vi "OnlyOpenTheseValves_CMD.vi"(11 "Valve List":u16[](array[numeric])) -> (3 "Valve Comand":T1)   [LabVIEW 2016]
panel:
  in  "Flowboard":enum16{"A", "B", "C"}(ring)
  in  "Channel":enum16{"1", "2", "3", "4", "5", "6", "7", "8"}(ring)
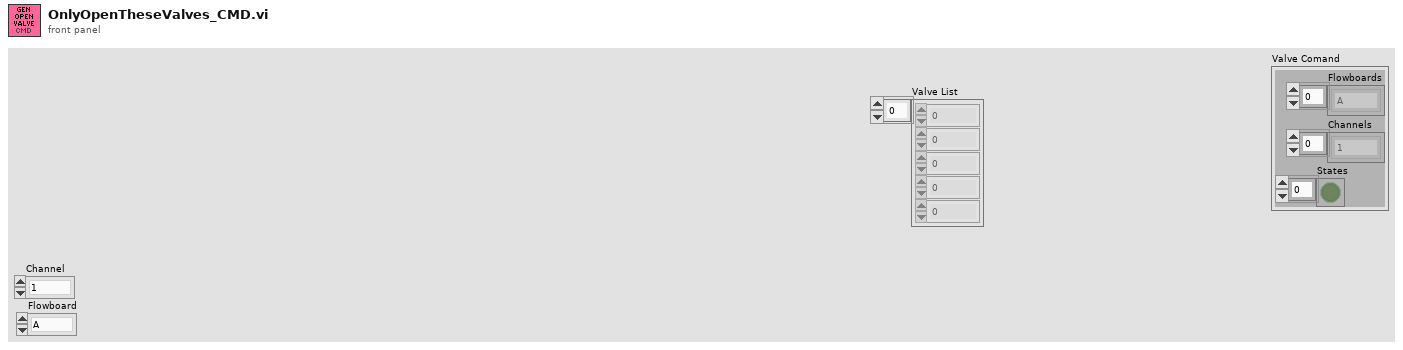
[diagram p1: front panel]
types:
  T1 = cluster{"Flowboards":enum16{"A", "B", "C"}[], "Channels":enum16{"1", "2", "3", "4", "5", "6", "7", "8"}[], "States":bool[]}
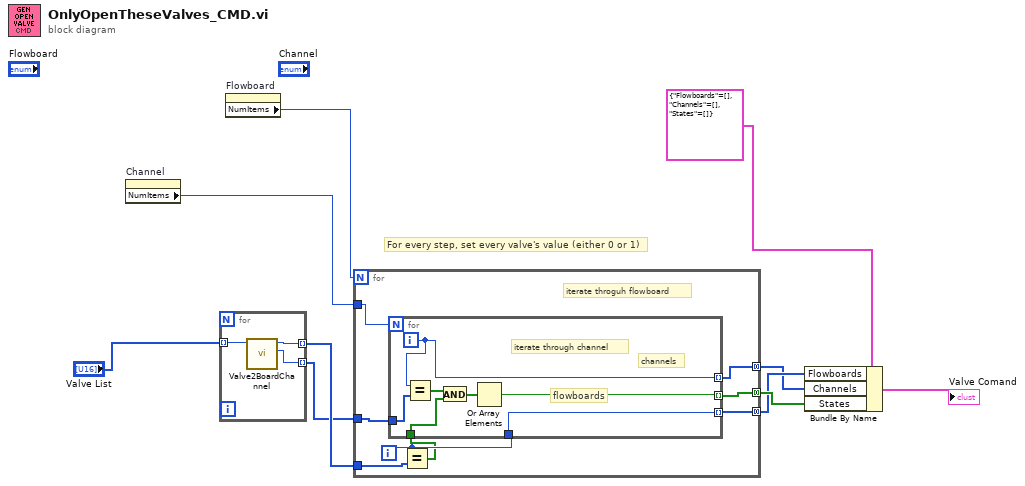
[diagram p0: block diagram]
diagram:
  # "For every step, set every valve's value (either 0 or 1)"
  n1 = property on="Channel" class="Enum (strict)"() -> ("NumItems"=w8:u32)  [unwired: 2 in, 2 out]
  n2 = for {
    tunnel: [w13] -> w4 mode=indexing
    tunnel: [w12] -> w3 mode=indexing
    tunnel: "Valve List" -> [w11] mode=indexing
    n3 = call "Valve2BoardChannel.vi"("ValveID"=w11) -> ("Channel"=w12:enum16{"1", "2", "3", "4", "5", "6", "7", "8"}, "Flowboard"=w13:enum16{"A", "B", "C"})  [unwired: 9 in]
  }
  n4 = property on="Flowboard" class="Enum (strict)"() -> ("NumItems"=w9:u32)  [unwired: 2 in, 2 out]
  n5 = for {
    N: w9 -> [_]
    tunnel: w8 -> [w21]
    tunnel: [w20] -> w5 mode=concatenating
    tunnel: [w19] -> w6 mode=concatenating
    tunnel: w4 -> [w17]
    tunnel: w3 -> [w18]
    tunnel: [w14] -> w7 mode=concatenating
    i -> [w16]
    # "iterate throguh flowboard"
    n6 = Equal?(x=w16, y=w17) -> (x = y?=w15:bool[])
    n7 = for {
      N: w21 -> [_]
      tunnel: [w27] -> w20 mode=indexing
      tunnel: w16 -> [w26]
      tunnel: [w26] -> w19 mode=indexing
      tunnel: w18 -> [w28]
      tunnel: w15 -> [w24]
      tunnel: [w22] -> w14 mode=indexing
      i -> [w27]
      # "flowboards"
      # "channels"
      # "iterate through channel"
      n8 = Equal?(x=w27, y=w28) -> (x = y?=w25:bool[])
      n9 = And(x=w25, y=w24) -> (x .and. y?=w23:bool[])
      n10 = Or Array Elements(Boolean array=w23) -> (logical OR=w22:bool)
    }
  }
  n11 = Bundle By Name(cluster=T1 {"Flowboards"=[], "Channels"=[], "States"=[]} ("Valve Data"), "Flowboards"=w6, "Channels"=w5, "States"=w7) -> (→"Valve Comand":T1)
